vi "Parse Error XML.vi"(9 "Code Tag Value":string, 10 "Error XML":string) -> (0 "Unknown Error":bool, 1 "Error Description Override":string, 2 "Error Code":i32, 3 "Warning":bool)   [LabVIEW 2015, in "NI_Azure_Core.lvlib"]
uses:
  NI_Azure_Core.lvlib
  XML Parsing/NI_Azure_XML Parsing.lvlib
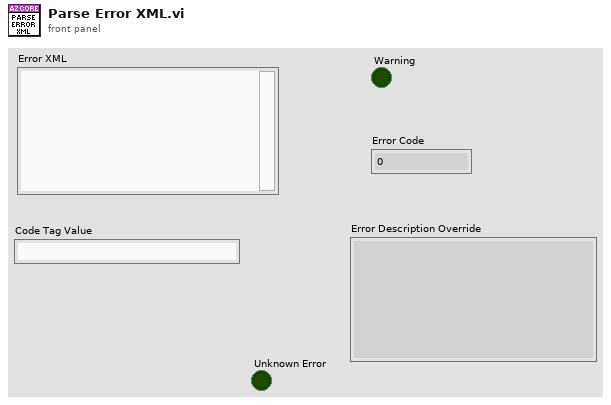
[diagram p1: front panel]
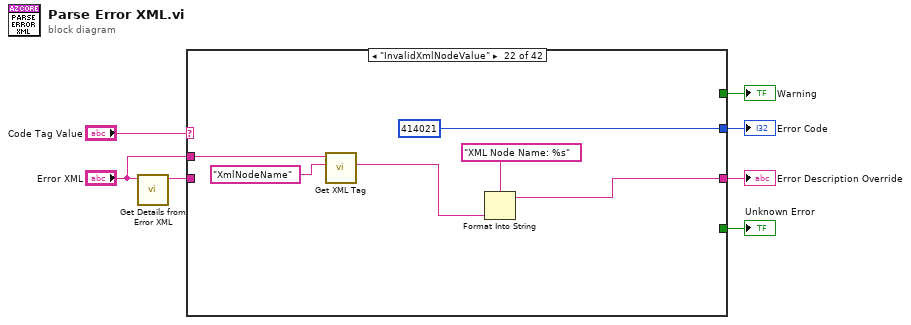
[diagram p0: block diagram]
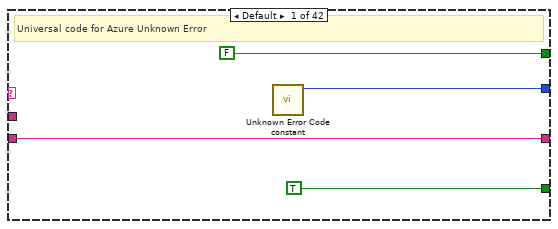
[diagram p2: hidden frame]
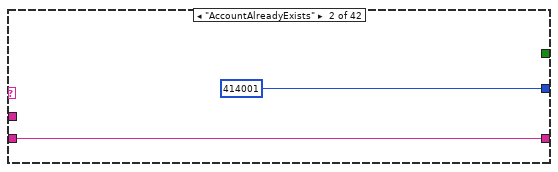
[diagram p3: hidden frame]
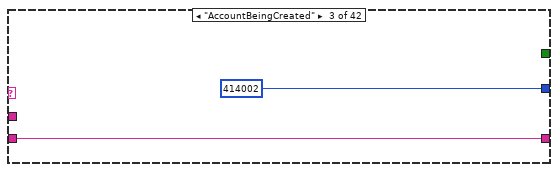
[diagram p4: hidden frame]
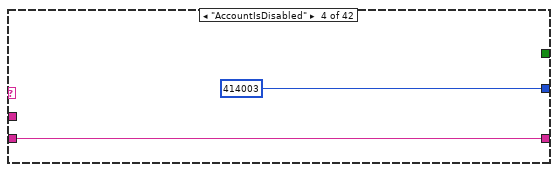
[diagram p5: hidden frame]
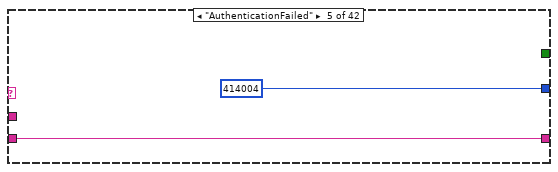
[diagram p6: hidden frame]
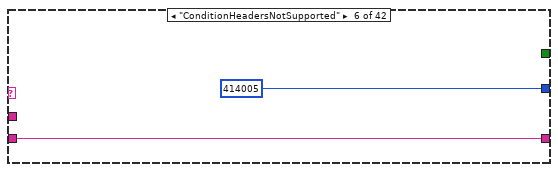
[diagram p7: hidden frame]
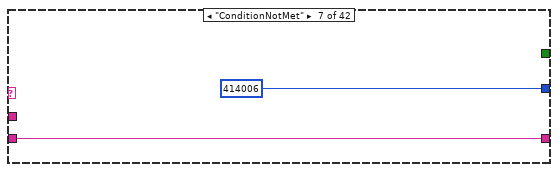
[diagram p8: hidden frame]
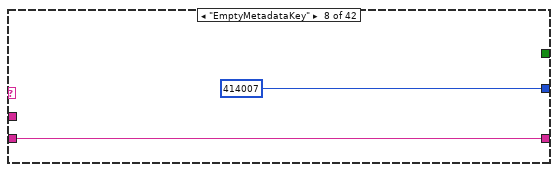
[diagram p9: hidden frame]
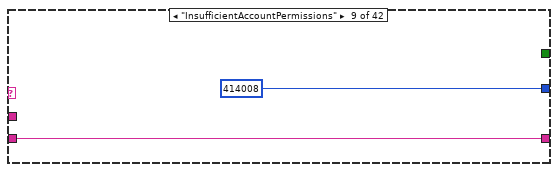
[diagram p10: hidden frame]
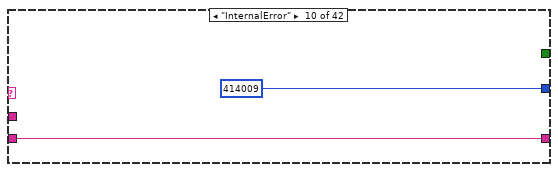
[diagram p11: hidden frame]
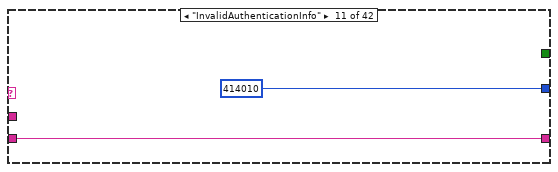
[diagram p12: hidden frame]
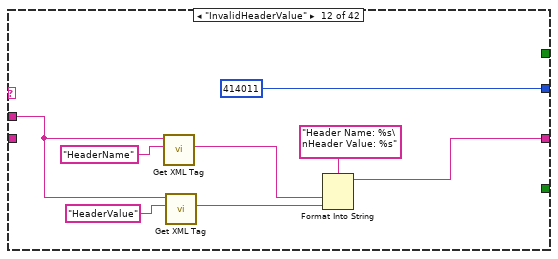
[diagram p13: hidden frame]
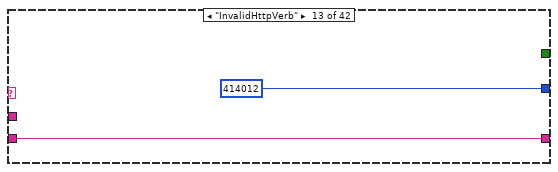
[diagram p14: hidden frame]
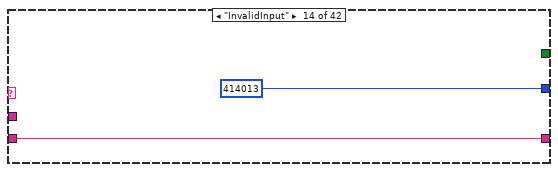
[diagram p15: hidden frame]
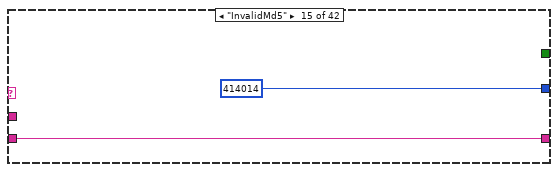
[diagram p16: hidden frame]
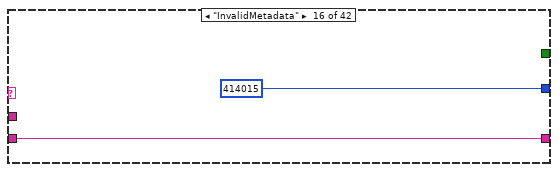
[diagram p17: hidden frame]
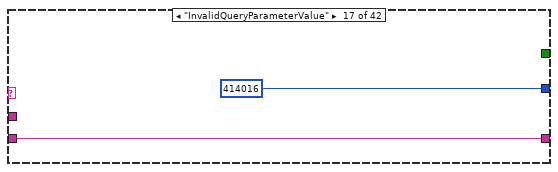
[diagram p18: hidden frame]
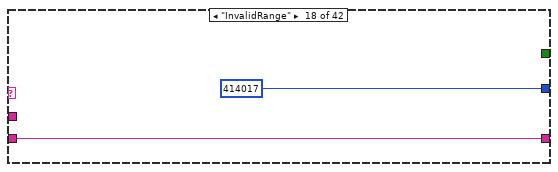
[diagram p19: hidden frame]
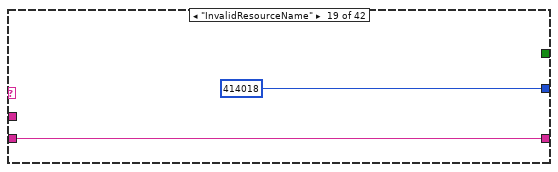
[diagram p20: hidden frame]
diagram:
  n1 = call "Get Details from Error XML.vi"("Error XML"="Error XML") -> ("Details"=w2:string)  [unwired: 10 in]
  n2 = case shown="\"InvalidXmlNodeValue\"" "Code Tag Value" {
    tunnel: [w10 414001 414002 414003 414004 414005 414006 414007 414008 414009 414010 414011 414012 414013 414014 414015 414016 414017 414018 414019 414020 414021 414022 414023 414024 414025 414026 414027 414028 414029 414030 414031 414032 414033 414034 414035 414036 414037 414038 414039 414040 414041] -> w5
    tunnel: [FALSE _ _ _ _ _ _ _ _ _ _ _ _ _ _ _ _ _ _ _ _ _ _ _ _ _ _ _ _ _ _ _ _ _ _ _ _ _ _ _ _ _] -> w6
    tunnel: w2 -> [w9 w12 w14 w16 w18 w20 w22 w24 w26 w28 w30 _ w40 w42 w44 w46 w48 w50 w52 w54 w56 _ w64 w66 w68 w70 w72 w74 w76 w78 w80 w82 w84 w86 w88 w90 w92 w94 w96 w98 w100 w102]
    tunnel: [w9 w12 w14 w16 w18 w20 w22 w24 w26 w28 w30 w33 w40 w42 w44 w46 w48 w50 w52 w54 w56 w58 w64 w66 w68 w70 w72 w74 w76 w78 w80 w82 w84 w86 w88 w90 w92 w94 w96 w98 w100 w102] -> w4
    tunnel: [TRUE _ _ _ _ _ _ _ _ _ _ _ _ _ _ _ _ _ _ _ _ _ _ _ _ _ _ _ _ _ _ _ _ _ _ _ _ _ _ _ _ _] -> w3
    tunnel: "Error XML" -> [_ _ _ _ _ _ _ _ _ _ _ w32 _ _ _ _ _ _ _ _ _ w59 _ _ _ _ _ _ _ _ _ _ _ _ _ _ _ _ _ _ _ _]
    frame Default {
      # "Universal code for Azure Unknown Error"
      n3 = call "Unknown Error Code constant.vi"() -> ("Azure Unknown Error Code value"=w10:i32)  [unwired: 11 in]
    }
    frame "AccountAlreadyExists" {
    }
    frame "AccountBeingCreated" {
    }
    frame "AccountIsDisabled" {
    }
    frame "AuthenticationFailed" {
    }
    frame "ConditionHeadersNotSupported" {
    }
    frame "ConditionNotMet" {
    }
    frame "EmptyMetadataKey" {
    }
    frame "InsufficientAccountPermissions" {
    }
    frame "InternalError" {
    }
    frame "InvalidAuthenticationInfo" {
    }
    frame "InvalidHeaderValue" {
      n4 = call "Get XML Tag.vi"("Tag name"="HeaderName", "XML String in"=w32) -> ("Tag value"=w35:string)  [unwired: 5 in, 4 out]
      n5 = call "Get XML Tag.vi"("Tag name"="HeaderValue", "XML String in"=w32) -> ("Tag value"=w34:string)  [unwired: 5 in, 4 out]
      n6 = Format Into String(format string="Header Name: %s\nHeader Value: %s", w35, w34) -> (resulting string=w33:string)  [unwired: 2 in, 1 out]
    }
    frame "InvalidHttpVerb" {
    }
    frame "InvalidInput" {
    }
    frame "InvalidMd5" {
    }
    frame "InvalidMetadata" {
    }
    frame "InvalidQueryParameterValue" {
    }
    frame "InvalidRange" {
    }
    frame "InvalidResourceName" {
    }
    frame "InvalidUri" {
    }
    frame "InvalidXmlDocument" {
    }
    frame "InvalidXmlNodeValue" {
      n7 = call "Get XML Tag.vi"("Tag name"="XmlNodeName", "XML String in"=w59) -> ("Tag value"=w60:string)  [unwired: 5 in, 4 out]
      n8 = Format Into String(format string="XML Node Name: %s", w60) -> (resulting string=w58:string)  [unwired: 2 in, 1 out]
    }
    frame "Md5Mismatch" {
    }
    frame "MetadataTooLarge" {
    }
    frame "MissingContentLengthHeader" {
    }
    frame "MissingRequiredQueryParameter" {
    }
    frame "MissingRequiredHeader" {
    }
    frame "MissingRequiredXmlNode" {
    }
    frame "MultipleConditionHeadersNotSupported" {
    }
    frame "OperationTimedOut" {
    }
    frame "OutOfRangeInput" {
    }
    frame "OutOfRangeQueryParameterValue" {
    }
    frame "RequestBodyTooLarge" {
    }
    frame "ResourceTypeMismatch" {
    }
    frame "RequestUrlFailedToParse" {
    }
    frame "ResourceAlreadyExists" {
    }
    frame "ResourceNotFound" {
    }
    frame "ServerBusy" {
    }
    frame "UnsupportedHeader" {
    }
    frame "UnsupportedXmlNode" {
    }
    frame "UnsupportedQueryParameter" {
    }
    frame "UnsupportedHttpVerb" {
    }
  }
  "Error Description Override" <- w4
  "Warning" <- w6
  "Error Code" <- w5
  "Unknown Error" <- w3
